vi "Check if Package Exists in SystemLink Feed.vi"(0 "SystemLink repo in":T1, 5 "feed name":string, 7 "package name":string, 9 "pacakge version":string, 11 "error in (no error)":errorcluster) -> (4 "SystemLink repo out":T1, 6 "feed name out":string, 8 "exists?":bool, 15 "error out":errorcluster)   [LabVIEW 2017, in "SystemLink_Repo_API.lvlib"]
doc: "Check if the specified package and version exists on the specified SystemLink feed."
uses:
  SystemLink_Repo_API.lvlib
  _support/systemlink repo.ctl
  <vilib>/httpClient/ClientHandle.ctl
  <vilib>/httpClient/LabVIEWHTTPClient.lvlib
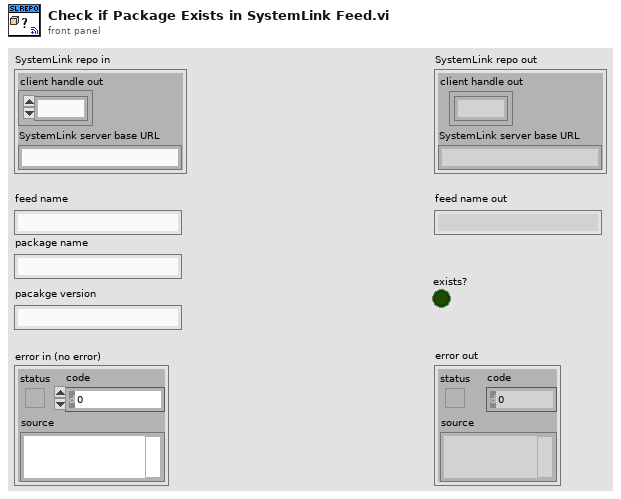
[diagram p1: front panel]
types:
  T1 = typedef "SystemLink_Repo_API.lvlib/systemlink repo.ctl" = cluster{"client handle out":T2, "SystemLink server base URL":string}
  T2 = typedef "LabVIEWHTTPClient.lvlib/ClientHandle.ctl" = refnum<k1>
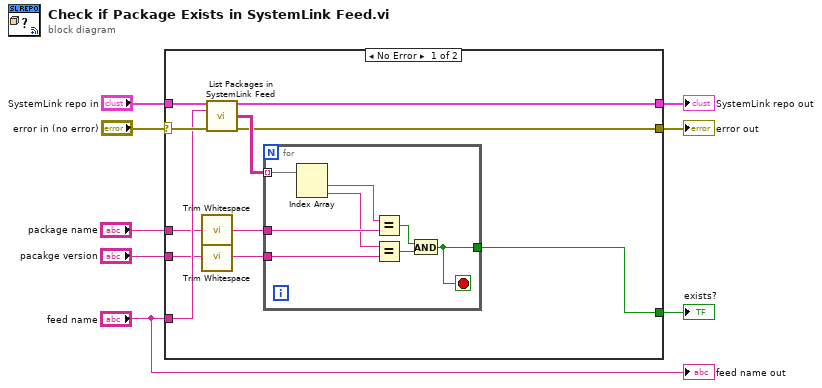
[diagram p0: block diagram]
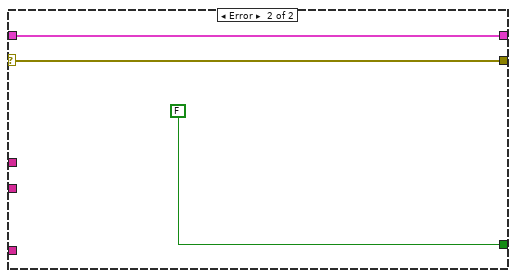
[diagram p2: hidden frame]
diagram:
  n1 = case shown="No Error" "error in (no error)" {
    selector: "error in (no error)" -> [w17 w30]
    tunnel: "SystemLink repo in" -> [w19 w29]
    tunnel: [w9 w30] -> w6
    tunnel: [w18 w29] -> w5
    tunnel: "feed name" -> [w16 _]
    tunnel: [w10 FALSE ("timed out?")] -> w3
    tunnel: "package name" -> [w14 _]
    tunnel: "pacakge version" -> [w13 _]
    frame No Error {
      n2 = call <vilib>:"Trim Whitespace.vi"("string"=w14) -> ("trimmed string"=w12:string)  [unwired: 1 in]
      n3 = call <vilib>:"Trim Whitespace.vi"("string"=w13) -> ("trimmed string"=w11:string)  [unwired: 1 in]
      n4 = call "List Packages in SystemLink Feed.vi"("SystemLink repo in"=w19, "feed name in"=w16, "error in (no error)"=w17) -> ("SystemLink repo out"=w18:T1, "packages"=w15:string[][], "error out"=w9:errorcluster)  [unwired: 9 in, 1 out]
      n5 = for {
        tunnel: w15 -> [w27] mode=indexing
        tunnel: w12 -> [w25]
        tunnel: w11 -> [w23]
        tunnel: [w20] -> w10
        stop <- w20 stop-if-true
        n6 = Index Array(array=w27) -> (element #1=w26:string, element #2=w24:string)  [unwired: 2 in]
        n7 = Equal?(x=w26, y=w25) -> (x = y?=w22:bool)
        n8 = Equal?(x=w24, y=w23) -> (x = y?=w21:bool)
        n9 = And(x=w22, y=w21) -> (x .and. y?=w20:bool)
      }
    }
    frame Error {
    }
  }
  "error out" <- w6
  "SystemLink repo out" <- w5
  "exists?" <- w3
  "feed name out" <- "feed name"
